vi "VI Tree.vi"   [LabVIEW 2018, in "OXYGEN.lvlib"]
uses:
  OXYGEN.lvlib
  Recording Control/SubVIs/RecordingControl_Start.vi
  Recording Control/SubVIs/RecordingControl_SetFileName.vi
  Measurement Values/SubVIs/AggregationRate_Set.vi
  Measurement Values/SubVIs/MeasurementItems_SetSingleChannel.vi
  Recording Control/SubVIs/RecordingControl_GetState.vi
  Recording Control/SubVIs/RecordingControl_Pause.vi
  Recording Control/SubVIs/RecordingControl_Stop.vi
  External Data Logging/SubVIs/ELOG_AggregationPeriod_Set.vi
  External Data Logging/SubVIs/ELOG_Calculations_Set.vi
  External Data Logging/SubVIs/ELOG_Channels_Set.vi
  External Data Logging/SubVIs/ELOG_Control_Start.vi
  External Data Logging/SubVIs/ELOG_OutputFormat_Set.vi
  External Data Logging/SubVIs/ELOG_TimestampFormat_Set.vi
  External Data Logging/SubVIs/ELOG_Control_Stop.vi
  Channel List Access/SubVIs/ChannelList_Attributes_GetProperty.vi
  Channel List Access/SubVIs/ChannelList_GetNames.vi
  Acquisition Control/SubVis/AcquisitionControl_Stop.vi
  Acquisition Control/SubVis/AcquisitionControl_Start.vi
  Application Control/SubVIs/ApplicationSetup_Load.vi
  Application Control/SubVIs/SystemTime_GetDate.vi
  Application Control/SubVIs/ScreenLock_SetLockState.vi
  Application Control/SubVIs/CommunicationFormat_SetActivationOutputHeader.vi
  Common Commands/SubVIs/ServiceRegister_Set.vi
  Common Commands/SubVIs/EventRegister_Clear.vi
  Common Commands/SubVIs/GetID.vi
  Error Handling/SubVIs/ErrorHandling_GetError.vi
  Error Handling/SubVIs/ErrorHandling_Range_Delete.vi
panel:
  # "SEE DIAGRAM\nFOR VI Tree"
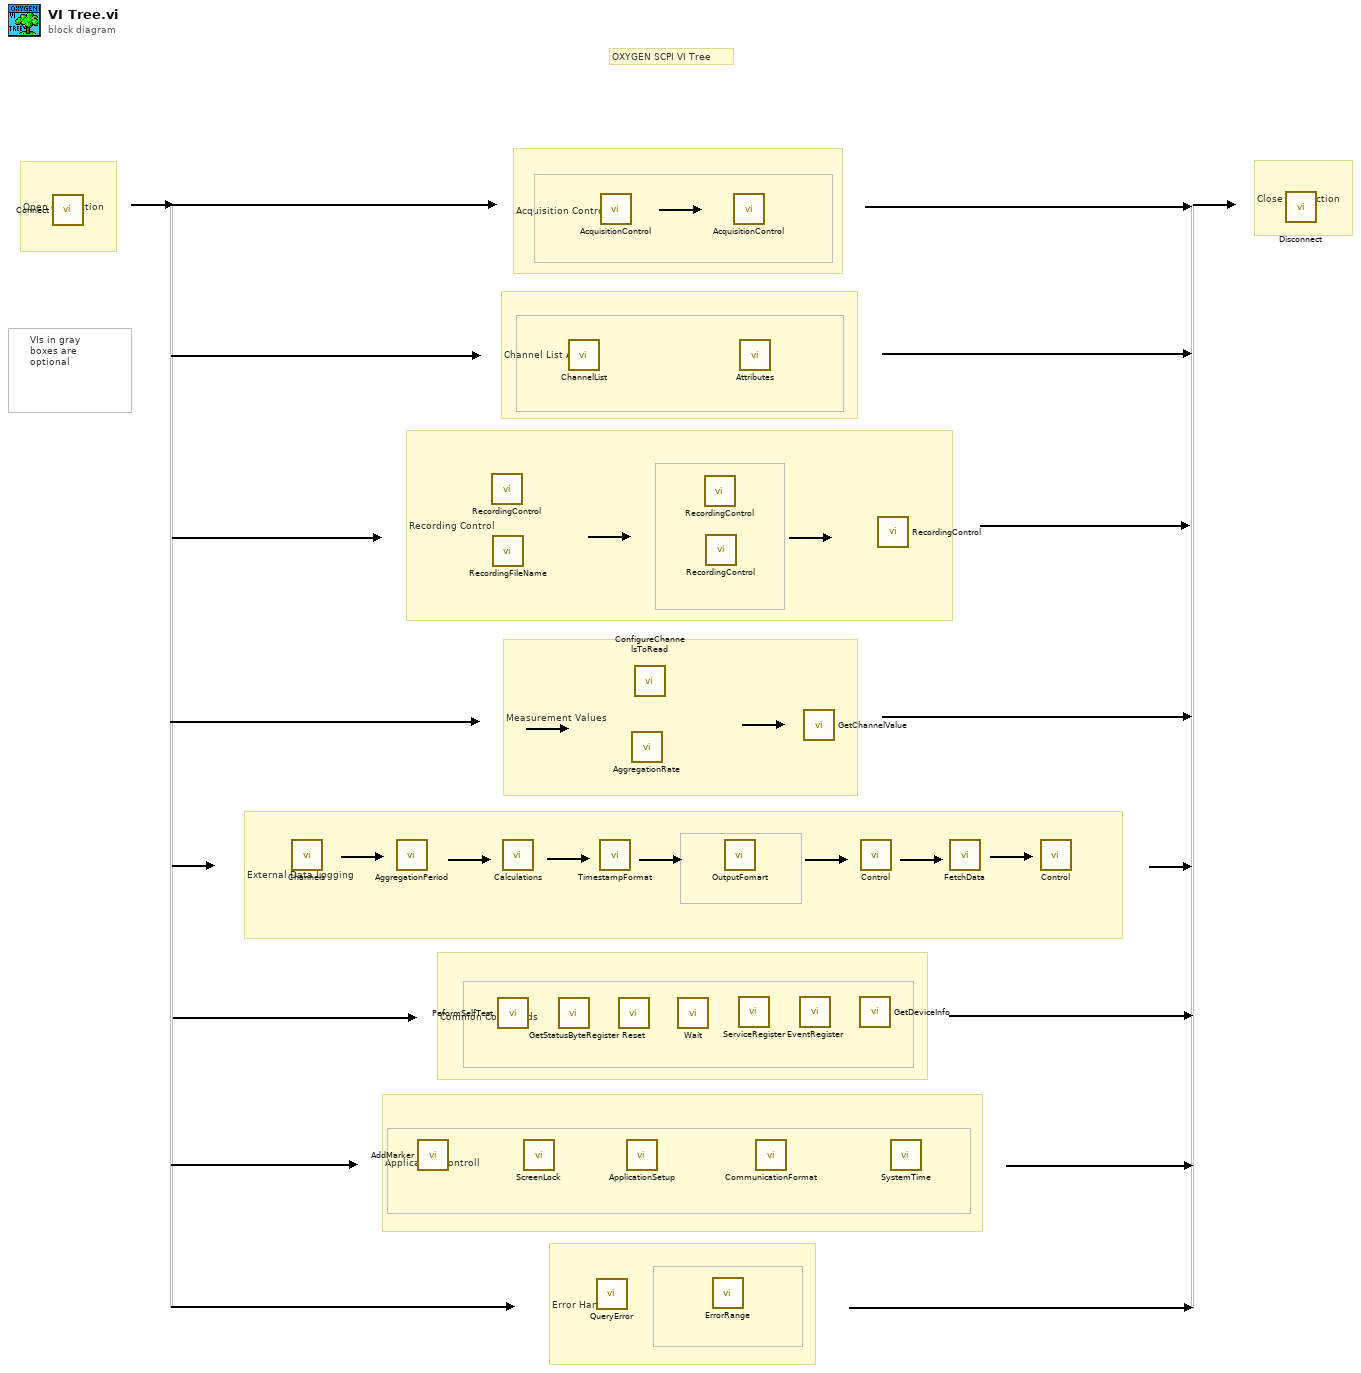
[diagram p0: block diagram]
diagram:
  # "VIs in gray\nboxes are\noptional"
  # "OXYGEN SCPI VI Tree"
  # "External Data Logging"
  # "Measurement Values"
  # "Recording Control"
  # "Common Commands"
  # "Channel List Access"
  # "Acquisition Control"
  # "Application Controll"
  # "Open connection"
  # "Error Handling"
  # "Close Connection"
  n1 = call "Connect.vi"() -> ()  [unwired: 10 in, 2 out]
  n2 = call-poly "Channels.vi"() -> ()  [unwired: 9 in, 3 out]
  n3 = call-poly "AggregationPeriod.vi"() -> ()  [unwired: 9 in, 3 out]
  n4 = call "AddMarker.vi"() -> ()  [unwired: 9 in, 3 out]
  n5 = call-poly "RecordingControl.vi"() -> ()  [unwired: 9 in, 3 out]
  n6 = call-poly "RecordingFileName.vi"() -> ()  [unwired: 9 in, 3 out]
  n7 = call "PeformSelfTest.vi"() -> ()  [unwired: 8 in, 4 out]
  n8 = call-poly "Calculations.vi"() -> ()  [unwired: 9 in, 3 out]
  n9 = call-poly "ScreenLock.vi"() -> ()  [unwired: 9 in, 3 out]
  n10 = call "GetStatusByteRegister.vi"() -> ()  [unwired: 8 in, 4 out]
  n11 = call-poly "ChannelList.vi"() -> ()  [unwired: 8 in, 4 out]
  n12 = call-poly "QueryError.vi"() -> ()  [unwired: 8 in, 4 out]
  n13 = call-poly "TimestampFormat.vi"() -> ()  [unwired: 9 in, 3 out]
  n14 = call-poly "AcquisitionControl.vi"() -> ()  [unwired: 9 in, 3 out]
  n15 = call "Reset.vi"() -> ()  [unwired: 9 in, 3 out]
  n16 = call-poly "ApplicationSetup.vi"() -> ()  [unwired: 9 in, 3 out]
  n17 = call-poly "AggregationRate.vi"() -> ()  [unwired: 9 in, 3 out]
  n18 = call-poly "ConfigureChannelsToRead.vi"() -> ()  [unwired: 9 in, 3 out]
  n19 = call "Wait.vi"() -> ()  [unwired: 9 in, 3 out]
  n20 = call-poly "RecordingControl.vi"() -> ()  [unwired: 9 in, 3 out]
  n21 = call-poly "RecordingControl.vi"() -> ()  [unwired: 8 in, 4 out]
  n22 = call-poly "ErrorRange.vi"() -> ()  [unwired: 9 in, 3 out]
  n23 = call-poly "OutputFomart.vi"() -> ()  [unwired: 9 in, 3 out]
  n24 = call-poly "AcquisitionControl.vi"() -> ()  [unwired: 9 in, 3 out]
  n25 = call-poly "ServiceRegister.vi"() -> ()  [unwired: 9 in, 3 out]
  n26 = call-poly "Attributes.vi"() -> ()  [unwired: 8 in, 4 out]
  n27 = call-poly "CommunicationFormat.vi"() -> ()  [unwired: 9 in, 3 out]
  n28 = call-poly "EventRegister.vi"() -> ()  [unwired: 9 in, 3 out]
  n29 = call "GetChannelValue.vi"() -> ()  [unwired: 8 in, 4 out]
  n30 = call-poly "GetDeviceInfo.vi"() -> ()  [unwired: 8 in, 4 out]
  n31 = call-poly "Control.vi"() -> ()  [unwired: 9 in, 3 out]
  n32 = call-poly "RecordingControl.vi"() -> ()  [unwired: 9 in, 3 out]
  n33 = call-poly "SystemTime.vi"() -> ()  [unwired: 8 in, 4 out]
  n34 = call "FetchData.vi"() -> ()  [unwired: 8 in, 4 out]
  n35 = call-poly "Control.vi"() -> ()  [unwired: 9 in, 3 out]
  n36 = call "Disconnect.vi"() -> ()  [unwired: 11 in, 1 out]
